vi "Stop Core.vi"(10 "final error code":i32, 11 "SAS_AFTester_Template in":refnum<class "Business Logic Tester.lvclass">) -> (3 "SAS_AFTester_Template out":refnum<class "Business Logic Tester.lvclass">)   [LabVIEW 2020, in "Business Logic Tester.lvlib" / "Business Logic Tester.lvclass"]
doc: "(<B>Filename</B>: Actor Framework.lvlib:Actor.lvclass:Stop Core.vi)\n\nDefines what the actor does before it stops. Use the <B>final error code</B> input to determine whether the actor shut down in response to an error.\n\nBy default, this method does nothing. A descendant class may override it to define behavior, such as shutting down any processes the actor initiated in its override of the Actor Core method."
uses:
  Business Logic Tester.lvclass
  Business Logic Tester.lvclass/Business Logic Tester.ctl
  <vilib>/ActorFramework/Actor/Actor.lvclass
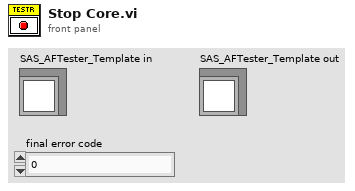
[diagram p1: front panel]
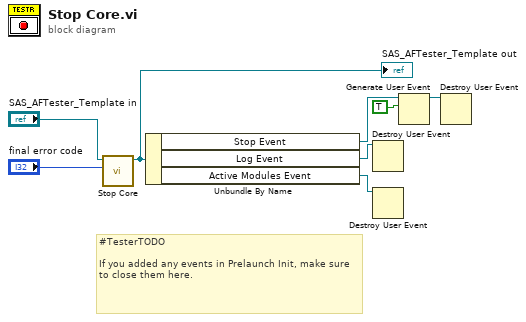
[diagram p0: block diagram]
diagram:
  # "#TesterTODO\n\nIf you added any events in Prelaunch Init, make sure to close them here."
  n1 = call-parent "Stop Core.vi"("final error code"="final error code", "Actor in"="SAS_AFTester_Template in") -> ("Actor out"=w6:refnum<class "Business Logic Tester.lvclass">)  [unwired: 9 in]
  "SAS_AFTester_Template out" <- w6
  n2 = Unbundle By Name(w6) -> ("Stop Event"=w4:refnum<user-event>, "Log Event"=w2:refnum<user-event>, "Active Modules Event"=w1:refnum<user-event>)
  n3 = Destroy User Event(user event=w2) -> ()  [unwired: 1 in, 1 out]
  n4 = Destroy User Event(user event=w1) -> ()  [unwired: 1 in, 1 out]
  n5 = Generate User Event(user event=w4, event data cluster=TRUE ("event data")) -> (user event out=w5:refnum<user-event>)  [unwired: 2 in, 1 out]
  n6 = Destroy User Event(user event=w5) -> ()  [unwired: 1 in, 1 out]
